vi "CRYBackup Work State.vi"   [LabVIEW 2013]
uses:
  CRYHardware Global.vi
panel:
  # "Backup Hardware Work State"
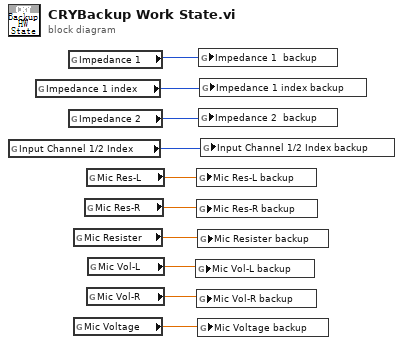
[diagram p0: block diagram]
diagram:
  n1 = global read "CRYHardware Global.vi" "Input Channel 1/2 Index"() -> (w7:i32)
  n2 = global read "CRYHardware Global.vi" "Impedance 1 index"() -> (w9:i32)
  n3 = global read "CRYHardware Global.vi" "Impedance 1"() -> (w10:i32)
  n4 = global read "CRYHardware Global.vi" "Impedance 2"() -> (w8:i32)
  n5 = global read "CRYHardware Global.vi" "Mic Resister"() -> (w4:dbl)
  n6 = global read "CRYHardware Global.vi" "Mic Voltage"() -> (w1:dbl)
  n7 = global read "CRYHardware Global.vi" "Mic Res-R"() -> (w5:dbl)
  n8 = global read "CRYHardware Global.vi" "Mic Res-L"() -> (w6:dbl)
  n9 = global read "CRYHardware Global.vi" "Mic Vol-R"() -> (w2:dbl)
  n10 = global read "CRYHardware Global.vi" "Mic Vol-L"() -> (w3:dbl)
  n11 = global write "CRYHardware Global.vi" "Mic Vol-L backup"(w3) -> ()
  n12 = global write "CRYHardware Global.vi" "Mic Res-L backup"(w6) -> ()
  n13 = global write "CRYHardware Global.vi" "Mic Res-R backup"(w5) -> ()
  n14 = global write "CRYHardware Global.vi" "Mic Vol-R backup"(w2) -> ()
  n15 = global write "CRYHardware Global.vi" "Mic Resister backup"(w4) -> ()
  n16 = global write "CRYHardware Global.vi" "Mic Voltage backup"(w1) -> ()
  n17 = global write "CRYHardware Global.vi" "Impedance 1  backup"(w10) -> ()
  n18 = global write "CRYHardware Global.vi" "Impedance 2  backup"(w8) -> ()
  n19 = global write "CRYHardware Global.vi" "Impedance 1 index backup"(w9) -> ()
  n20 = global write "CRYHardware Global.vi" "Input Channel 1/2 Index backup"(w7) -> ()
